vi "Build_Filename_with_Date_Time.vi"(9 "File Extension (.csv)":string=".csv", 10 "Filename Prefix":string, 11 "Folder for Data Captures":path) -> (3 "File Path Output":string)   [LabVIEW 2023]
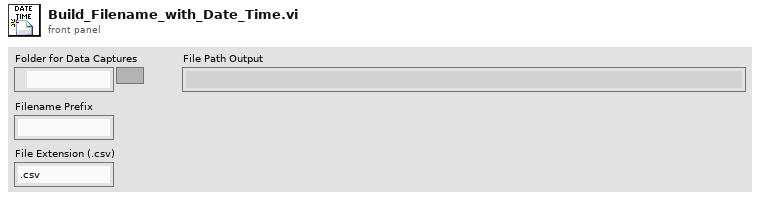
[diagram p1: front panel]
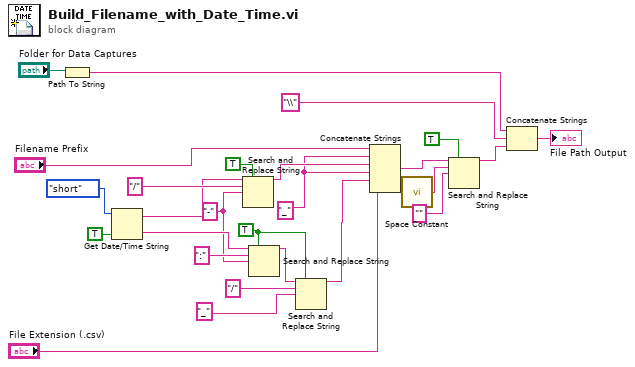
[diagram p0: block diagram]
diagram:
  w10 = "_" ("replace string (\"\")")
  w17 = TRUE ("replace all? (F)")
  w13 = "-" ("replace string (\"\")")
  n1 = Path To String(path="Folder for Data Captures") -> (string=w2:string)
  n2 = Get Date/Time String(date format (0)=enum16{"short", "long", "abbreviated"}."short", want seconds? (F)=TRUE) -> (date string=w14:string, time string=w22:string)  [unwired: 1 in]
  n3 = Search and Replace String(replace all?=TRUE ("replace all? (F)"), input string=w14, search string="/" ("replace string (\"\")"), replace string=w13) -> (result string=w11:string)  [unwired: 4 in, 3 out]
  n4 = Search and Replace String(replace all?=w17, input string=w22, search string=":" ("replace string (\"\")"), replace string=w13) -> (result string=w19:string)  [unwired: 4 in, 3 out]
  n5 = Search and Replace String(replace all?=w17, input string=w19, search string="/" ("replace string (\"\")"), replace string="_" ("replace string (\"\")")) -> (result string=w18:string)  [unwired: 4 in, 3 out]
  n6 = Concatenate Strings("Filename Prefix", w10, w11, w10, w18, "File Extension (.csv)") -> (w9:string)
  n7 = call <vilib>:"Space Constant.vi"() -> ("String"=w7:string)
  n8 = Search and Replace String(replace all?=TRUE ("replace all? (F)"), input string=w9, search string=w7, replace string="" ("replace string (\"\")")) -> (result string=w5:string)  [unwired: 4 in, 3 out]
  n9 = Concatenate Strings(w2, "\\" ("string"), w5) -> (→"File Path Output":string)
